vi "Configure Null.vi"(8 "error in (no error)":errorcluster, 11 "8846A in":refnum<class "8846A.lvclass">) -> (0 "error out":errorcluster, 3 "8846A out":refnum<class "8846A.lvclass">)   [LabVIEW 2015, in "8846A.lvclass"]
uses:
  8846A.lvclass
  <instrlib>/Fluke 884X Series/Fluke 884X Series.lvlib
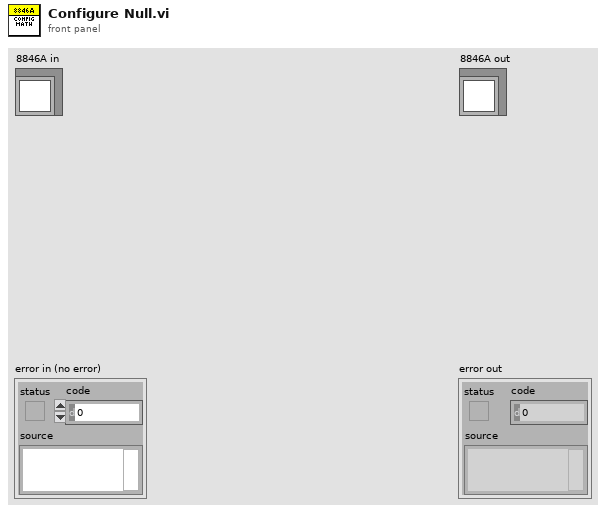
[diagram p1: front panel]
types:
  T1 = enum16{"None", "Min/Max", "Null", "dB", "dBm", "Limit"}
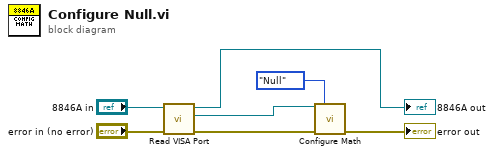
[diagram p0: block diagram]
diagram:
  n1 = call-dynamic "Read VISA Port.vi"("error in (no error)"="error in (no error)", "Device in"="8846A in") -> ("error out"=w2:errorcluster, "VISA Port"=w4:refnum<visa-resource-name>, "Device out"=→"8846A out":refnum<class "8846A.lvclass">)  [unwired: 7 in]
  n2 = call <instrlib>:"Configure Math.vi"("VISA resource name"=w4, "Operation (0:None)"=T1."Null", "error in (no error)"=w2) -> ("error out"=→"error out":errorcluster)  [unwired: 11 in, 1 out]
